vi "Count Status.vi"(10 "Status":T1, 11 "Method Result in":refnum<class "Method Result.lvclass">) -> (2 "Count":i32, 3 "Method Result out":refnum<class "Method Result.lvclass">)   [LabVIEW 2020, in "Method Result.lvclass"]
uses:
  Method Result.lvclass
  Assertion Result/Assertion Result.lvclass
  Assertion Result/Public/TypeDefs/Status.ctl
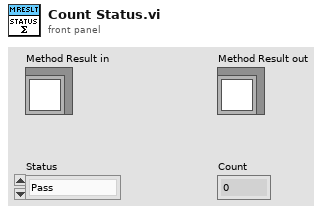
[diagram p1: front panel]
types:
  T1 = typedef "Assertion Result.lvclass/Status.ctl" = enum16{"Pass", "Fail", "Error", "Skipped", "Setup Error", "Broken", "Teardown Error"}
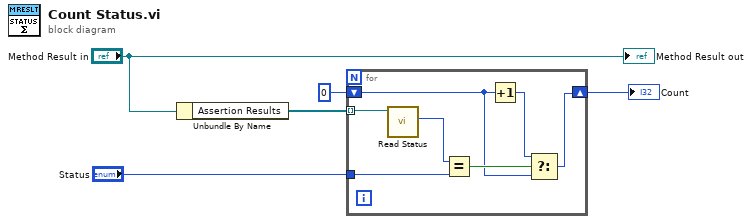
[diagram p0: block diagram]
diagram:
  n1 = Unbundle By Name("Method Result in") -> ("Assertion Results"=w4:refnum<class "Assertion Result.lvclass">[])
  n2 = for {
    tunnel: w4 -> [w12] mode=indexing
    shift-right: [w7] -> w3
    shift-left: 0 -> [w8]
    tunnel: "Status" -> [w6]
    n3 = call "Read Status.vi"("Assertion Result In"=w12) -> ("Status"=w11:T1)  [unwired: 9 in, 1 out]
    n4 = Equal?(x=w11, y=w6) -> (x = y?=w10:bool)
    n5 = Increment(x=w8) -> (x+1=w9:i32)
    n6 = Select(t=w9, s=w10, f=w8) -> (s? t:f=w7:i32)
  }
  "Count" <- w3
  "Method Result out" <- "Method Result in"
